vi "VideoMux Base URL Const.vi"() -> (2 "VideoMux Base URL":string="http://192.168.42.138")   [LabVIEW 2022 SP3, in "TouchControl.lvlib"]
uses:
  TouchControl.lvlib
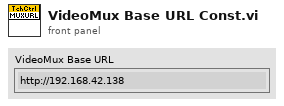
[diagram p1: front panel]
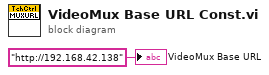
[diagram p0: block diagram]
diagram:
  "VideoMux Base URL" <- "http://192.168.42.138"
